vi "State_Waiting.vi"(8 "error in (no error)":T1, 9 "Parameter":variant, 10 "Command":string, 11 "Sim DiscreteIO in":class) -> (0 "error out":T1, 2 "Debug Message":string, 3 "Sim DiscreteIO out":class)   [LabVIEW 2021, in "Sim DiscreteIO.lvclass"]
uses:
  Sim DiscreteIO.lvclass
  C:/Program Files (x86)/National Instruments/LabVIEW 2021/user.lib/S2 Labs/Module Framework/Modules/Base/Module.lvclass
  Sim DiscreteIO.lvclass/Sim DiscreteIO.ctl
  <userlib>/S2 Labs/Module Framework/Modules/Base/Module.lvclass/Module.ctl
  <userlib>/S2 Labs/CVT Toolkit/CVT.lvclass/CVT.ctl
  c5649ace-d903-4788-aea9-226f7769309e.vi
  82162073-8ea0-43ea-a5e7-9bcd401e2448.vi
  Accessors/Write Initialized.vi
  Accessors/Read ch_labels.vi
  Accessors/Read occurrence.vi
  82162073-8ea0-43ea-a5e7-9bcd401e2448.vi/71b19a30-41bb-452f-8775-2cd3e07414b9.vi
  <userlib>/S2 Labs/Module Framework/Modules/Base/Read Module CVT.vi
  <userlib>/S2 Labs/CVT Toolkit/Variant Functions/Write Reserved Attributes.vi
  <userlib>/S2 Labs/CVT Toolkit/Read CVT DVR.vi
  <userlib>/S2 Labs/CVT Toolkit/Variant Functions/Write Alias Attribute.vi
  <userlib>/S2 Labs/CVT Toolkit/Variant Functions/Write Unit Attribute.vi
  <userlib>/S2 Labs/CVT Toolkit/Variant Functions/Write Type Attribute.vi
  <userlib>/S2 Labs/CVT Toolkit/Variant Functions/Write Parms Attribute.vi
  <vilib>/Utility/error.llb/Error Cluster From Error Code.vi
  <vilib>/rvi/errors/niLvFpgaAdjustHostInterfaceError.vi
  <userlib>/S2 Labs/Module Framework/Modules/Base/Trigger Logging Write.vi
  <vilib>/rvi/interface/nirviReadWriteControl/nirviReadWriteControl.xnode
  <userlib>/S2 Labs/CVT Toolkit/CVT.lvclass
  <userlib>/S2 Labs/Module Framework/Modules/Base/Module.lvclass
  NiFpgaLv.dll
  <vilib>/rvi/interface/Simulation/niFpgaSimulationCallBeginRW.vi
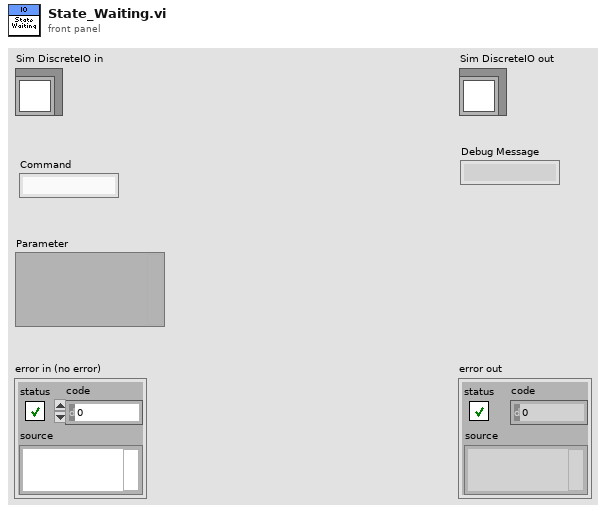
[diagram p1: front panel]
types:
  T1 = cluster{"source":string, "code":numeric, "status":boolean}
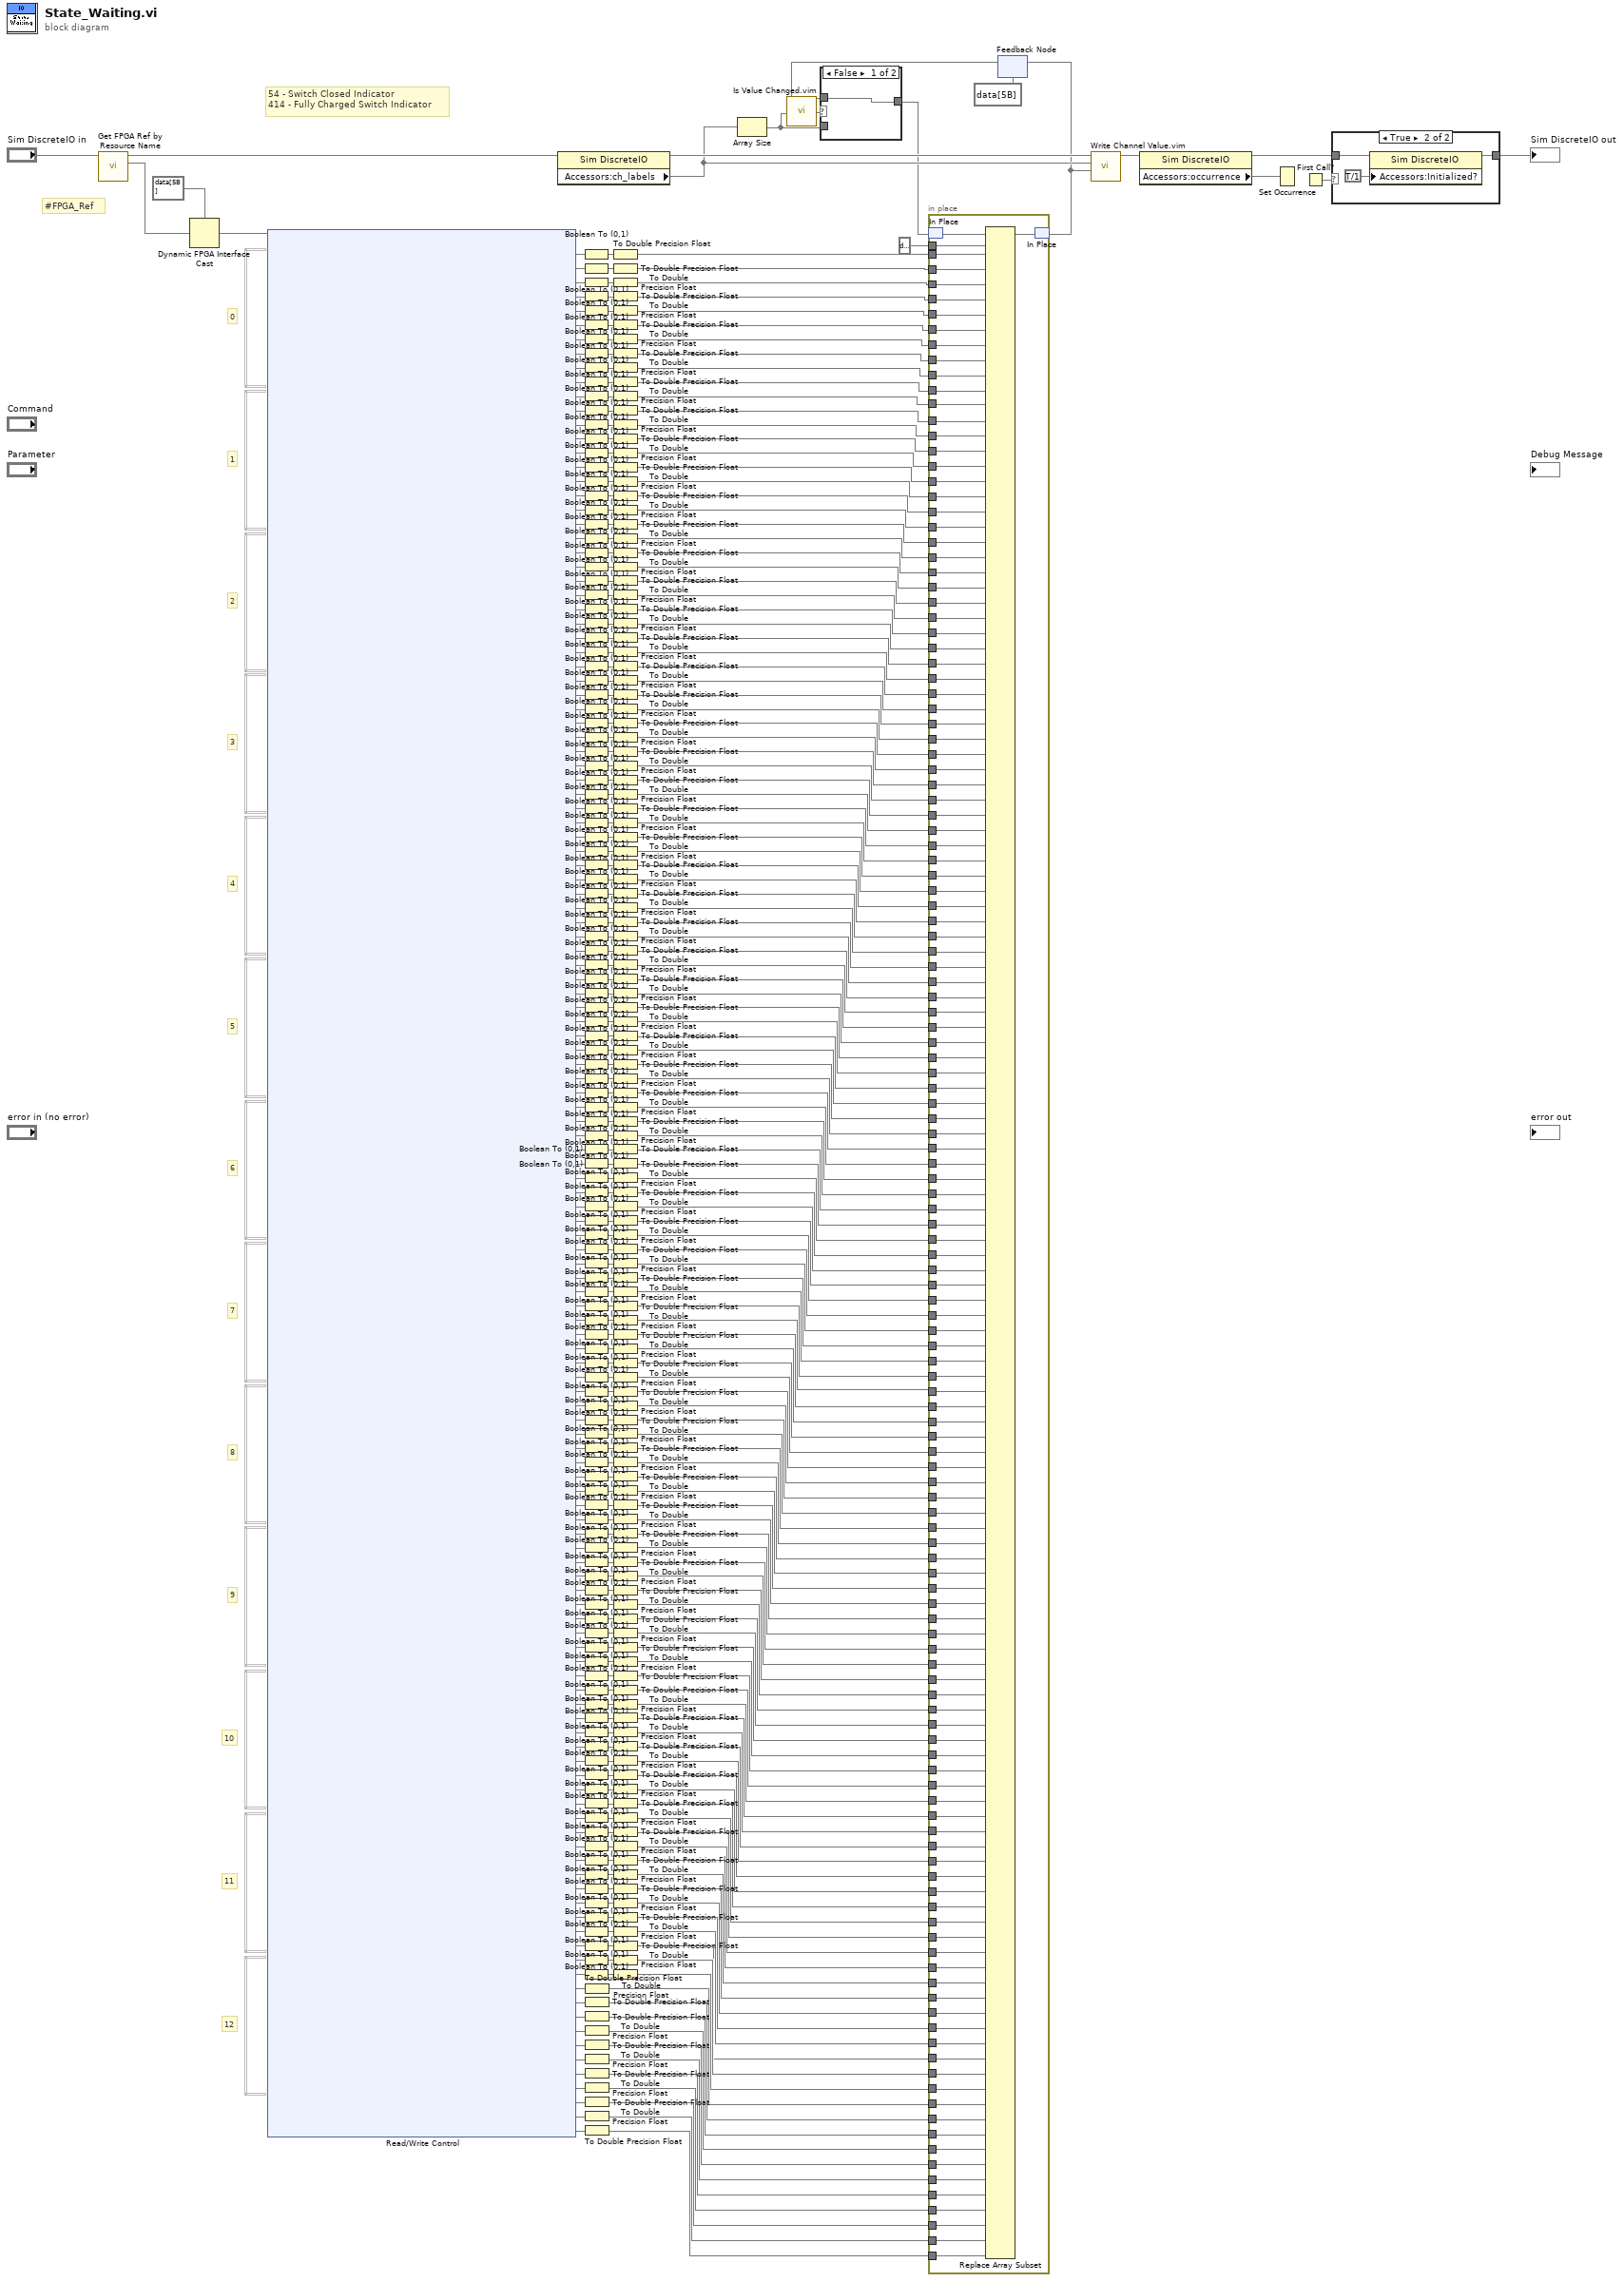
[diagram p0: block diagram]
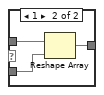
[diagram p2: hidden frame]
diagram:
  # "54 - Switch Closed Indicator\n414 - Fully Charged Switch Indicator"
  # "12"
  # "11"
  # "10"
  # "9"
  # "8"
  # "7"
  # "6"
  # "5"
  # "4"
  # "3"
  # "2"
  # "1"
  # "0"
  # "#FPGA_Ref"
  n1 = call <userlib>:"Get FPGA Ref by Resource Name.vi"(11:"Sim DiscreteIO in") -> (2:w405, 3:w12)  [unwired: 7 in, 2 out]
  n2 = Dynamic FPGA Interface Cast(Session In=data[5B] ("Type"), Type=w405) -> (Session Out=w17)
  n3 = xnode "Read/Write Control"(w17) -> (w20, w23, w26, w30, w35, w36, w37, w38, w44, w45, w57, w58, w59, w60, w61, w62, w63, w64, w65, w66, w86, w87, w88, w89, w90, w91, w92, w93, w94, w95, w115, w116, w117, w118, w119, w120, w121, w122, w123, w124, w148, w149, w150, w151, w152, w153, w154, w155, w156, w157, w178, w179, w180, w181, w182, w183, w184, w185, w186, w327, w328, w5, w4, w187, w208, w209, w210, w211, w212, w213, w214, w215, w216, w217, w238, w239, w240, w241, w242, w243, w244, w245, w246, w247, w267, w269, w270, w271, w272, w273, w274, w275, w276, w277, w296, w301, w302, w303, w330, w331, w304, w305, w333, w306, w307, w334, w345, w346, w351, w352, w357, w358, w364, w365, w366, w367, w379, w380, w381, w382, w383, w384, w312, w313, w314, w315, w316, w317, w318, w319, w320, w321, w322)  [unwired: 1 in, 2 out]
  n4 = property class="Sim DiscreteIO"(reference=w12) -> (reference out=w11, "Accessors:ch_labels"=w10)  [unwired: 1 in, 1 out]
  n5 = Boolean To (0,1)(Boolean=w20) -> (0, 1=w19)
  n6 = Boolean To (0,1)(Boolean=w23) -> (0, 1=w22)
  n7 = Boolean To (0,1)(Boolean=w26) -> (0, 1=w25)
  n8 = Boolean To (0,1)(Boolean=w30) -> (0, 1=w24)
  n9 = Boolean To (0,1)(Boolean=w35) -> (0, 1=w34)
  n10 = Boolean To (0,1)(Boolean=w36) -> (0, 1=w33)
  n11 = Boolean To (0,1)(Boolean=w37) -> (0, 1=w31)
  n12 = Boolean To (0,1)(Boolean=w38) -> (0, 1=w32)
  n13 = Boolean To (0,1)(Boolean=w44) -> (0, 1=w133)
  n14 = Boolean To (0,1)(Boolean=w45) -> (0, 1=w43)
  n15 = Boolean To (0,1)(Boolean=w57) -> (0, 1=w56)
  n16 = Boolean To (0,1)(Boolean=w58) -> (0, 1=w55)
  n17 = Boolean To (0,1)(Boolean=w59) -> (0, 1=w53)
  n18 = Boolean To (0,1)(Boolean=w60) -> (0, 1=w54)
  n19 = Boolean To (0,1)(Boolean=w61) -> (0, 1=w49)
  n20 = Boolean To (0,1)(Boolean=w62) -> (0, 1=w50)
  n21 = Boolean To (0,1)(Boolean=w63) -> (0, 1=w52)
  n22 = Boolean To (0,1)(Boolean=w64) -> (0, 1=w51)
  n23 = Boolean To (0,1)(Boolean=w65) -> (0, 1=w324)
  n24 = Boolean To (0,1)(Boolean=w66) -> (0, 1=w48)
  n25 = Boolean To (0,1)(Boolean=w86) -> (0, 1=w77)
  n26 = Boolean To (0,1)(Boolean=w87) -> (0, 1=w78)
  n27 = Boolean To (0,1)(Boolean=w88) -> (0, 1=w80)
  n28 = Boolean To (0,1)(Boolean=w89) -> (0, 1=w79)
  n29 = Boolean To (0,1)(Boolean=w90) -> (0, 1=w84)
  n30 = Boolean To (0,1)(Boolean=w91) -> (0, 1=w83)
  n31 = Boolean To (0,1)(Boolean=w92) -> (0, 1=w81)
  n32 = Boolean To (0,1)(Boolean=w93) -> (0, 1=w82)
  n33 = Boolean To (0,1)(Boolean=w94) -> (0, 1=w132)
  n34 = Boolean To (0,1)(Boolean=w95) -> (0, 1=w85)
  n35 = Boolean To (0,1)(Boolean=w115) -> (0, 1=w114)
  n36 = Boolean To (0,1)(Boolean=w116) -> (0, 1=w113)
  n37 = Boolean To (0,1)(Boolean=w117) -> (0, 1=w111)
  n38 = Boolean To (0,1)(Boolean=w118) -> (0, 1=w112)
  n39 = Boolean To (0,1)(Boolean=w119) -> (0, 1=w107)
  n40 = Boolean To (0,1)(Boolean=w120) -> (0, 1=w108)
  n41 = Boolean To (0,1)(Boolean=w121) -> (0, 1=w110)
  n42 = Boolean To (0,1)(Boolean=w122) -> (0, 1=w109)
  n43 = Boolean To (0,1)(Boolean=w123) -> (0, 1=w131)
  n44 = Boolean To (0,1)(Boolean=w124) -> (0, 1=w106)
  n45 = Boolean To (0,1)(Boolean=w148) -> (0, 1=w139)
  n46 = Boolean To (0,1)(Boolean=w149) -> (0, 1=w140)
  n47 = Boolean To (0,1)(Boolean=w150) -> (0, 1=w142)
  n48 = Boolean To (0,1)(Boolean=w151) -> (0, 1=w141)
  n49 = Boolean To (0,1)(Boolean=w152) -> (0, 1=w146)
  n50 = Boolean To (0,1)(Boolean=w153) -> (0, 1=w145)
  n51 = Boolean To (0,1)(Boolean=w154) -> (0, 1=w143)
  n52 = Boolean To (0,1)(Boolean=w155) -> (0, 1=w144)
  n53 = Boolean To (0,1)(Boolean=w156) -> (0, 1=w138)
  n54 = Boolean To (0,1)(Boolean=w157) -> (0, 1=w147)
  n55 = Boolean To (0,1)(Boolean=w178) -> (0, 1=w176)
  n56 = Boolean To (0,1)(Boolean=w179) -> (0, 1=w175)
  n57 = Boolean To (0,1)(Boolean=w180) -> (0, 1=w173)
  n58 = Boolean To (0,1)(Boolean=w181) -> (0, 1=w174)
  n59 = Boolean To (0,1)(Boolean=w182) -> (0, 1=w169)
  n60 = Boolean To (0,1)(Boolean=w183) -> (0, 1=w170)
  n61 = Boolean To (0,1)(Boolean=w184) -> (0, 1=w172)
  n62 = Boolean To (0,1)(Boolean=w185) -> (0, 1=w171)
  n63 = Boolean To (0,1)(Boolean=w186) -> (0, 1=w177)
  n64 = Boolean To (0,1)(Boolean=w327) -> (0, 1=w326)
  n65 = Boolean To (0,1)(Boolean=w328) -> (0, 1=w325)
  n66 = Boolean To (0,1)(Boolean=w5) -> (0, 1=w6)
  n67 = Boolean To (0,1)(Boolean=w4) -> (0, 1=w7)
  n68 = Boolean To (0,1)(Boolean=w187) -> (0, 1=w168)
  n69 = Boolean To (0,1)(Boolean=w208) -> (0, 1=w199)
  n70 = Boolean To (0,1)(Boolean=w209) -> (0, 1=w200)
  n71 = Boolean To (0,1)(Boolean=w210) -> (0, 1=w202)
  n72 = Boolean To (0,1)(Boolean=w211) -> (0, 1=w201)
  n73 = Boolean To (0,1)(Boolean=w212) -> (0, 1=w206)
  n74 = Boolean To (0,1)(Boolean=w213) -> (0, 1=w205)
  n75 = Boolean To (0,1)(Boolean=w214) -> (0, 1=w203)
  n76 = Boolean To (0,1)(Boolean=w215) -> (0, 1=w204)
  n77 = Boolean To (0,1)(Boolean=w216) -> (0, 1=w198)
  n78 = Boolean To (0,1)(Boolean=w217) -> (0, 1=w207)
  n79 = Boolean To (0,1)(Boolean=w238) -> (0, 1=w236)
  n80 = Boolean To (0,1)(Boolean=w239) -> (0, 1=w235)
  n81 = Boolean To (0,1)(Boolean=w240) -> (0, 1=w233)
  n82 = Boolean To (0,1)(Boolean=w241) -> (0, 1=w234)
  n83 = Boolean To (0,1)(Boolean=w242) -> (0, 1=w229)
  n84 = Boolean To (0,1)(Boolean=w243) -> (0, 1=w230)
  n85 = Boolean To (0,1)(Boolean=w244) -> (0, 1=w232)
  n86 = Boolean To (0,1)(Boolean=w245) -> (0, 1=w231)
  n87 = Boolean To (0,1)(Boolean=w246) -> (0, 1=w237)
  n88 = Boolean To (0,1)(Boolean=w247) -> (0, 1=w228)
  n89 = Boolean To (0,1)(Boolean=w267) -> (0, 1=w268)
  n90 = Boolean To (0,1)(Boolean=w269) -> (0, 1=w259)
  n91 = Boolean To (0,1)(Boolean=w270) -> (0, 1=w261)
  n92 = Boolean To (0,1)(Boolean=w271) -> (0, 1=w260)
  n93 = Boolean To (0,1)(Boolean=w272) -> (0, 1=w265)
  n94 = Boolean To (0,1)(Boolean=w273) -> (0, 1=w264)
  n95 = Boolean To (0,1)(Boolean=w274) -> (0, 1=w262)
  n96 = Boolean To (0,1)(Boolean=w275) -> (0, 1=w263)
  n97 = Boolean To (0,1)(Boolean=w276) -> (0, 1=w258)
  n98 = Boolean To (0,1)(Boolean=w277) -> (0, 1=w266)
  n99 = Boolean To (0,1)(Boolean=w296) -> (0, 1=w288)
  n100 = Boolean To (0,1)(Boolean=w301) -> (0, 1=w294)
  n101 = Boolean To (0,1)(Boolean=w302) -> (0, 1=w292)
  n102 = Boolean To (0,1)(Boolean=w303) -> (0, 1=w293)
  n103 = Boolean To (0,1)(Boolean=w330) -> (0, 1=w329)
  n104 = Boolean To (0,1)(Boolean=w331) -> (0, 1=w341)
  n105 = Boolean To (0,1)(Boolean=w304) -> (0, 1=w290)
  n106 = Boolean To (0,1)(Boolean=w305) -> (0, 1=w291)
  n107 = Boolean To (0,1)(Boolean=w333) -> (0, 1=w332)
  n108 = Boolean To (0,1)(Boolean=w306) -> (0, 1=w295)
  n109 = Boolean To (0,1)(Boolean=w307) -> (0, 1=w289)
  n110 = Boolean To (0,1)(Boolean=w334) -> (0, 1=w342)
  n111 = Boolean To (0,1)(Boolean=w345) -> (0, 1=w344)
  n112 = Boolean To (0,1)(Boolean=w346) -> (0, 1=w343)
  n113 = Boolean To (0,1)(Boolean=w351) -> (0, 1=w349)
  n114 = Boolean To (0,1)(Boolean=w352) -> (0, 1=w350)
  n115 = Boolean To (0,1)(Boolean=w357) -> (0, 1=w356)
  n116 = Boolean To (0,1)(Boolean=w358) -> (0, 1=w355)
  n117 = Boolean To (0,1)(Boolean=w364) -> (0, 1=w372)
  n118 = Boolean To (0,1)(Boolean=w365) -> (0, 1=w363)
  n119 = Boolean To (0,1)(Boolean=w366) -> (0, 1=w361)
  n120 = Boolean To (0,1)(Boolean=w367) -> (0, 1=w362)
  n121 = Boolean To (0,1)(Boolean=w379) -> (0, 1=w377)
  n122 = Boolean To (0,1)(Boolean=w380) -> (0, 1=w378)
  n123 = Boolean To (0,1)(Boolean=w381) -> (0, 1=w373)
  n124 = Boolean To (0,1)(Boolean=w382) -> (0, 1=w374)
  n125 = Boolean To (0,1)(Boolean=w383) -> (0, 1=w376)
  n126 = Boolean To (0,1)(Boolean=w384) -> (0, 1=w375)
  n127 = To Double Precision Float(number=w312) -> (double precision float=w391)
  n128 = To Double Precision Float(number=w313) -> (double precision float=w392)
  n129 = To Double Precision Float(number=w314) -> (double precision float=w393)
  n130 = To Double Precision Float(number=w315) -> (double precision float=w394)
  n131 = To Double Precision Float(number=w316) -> (double precision float=w395)
  n132 = To Double Precision Float(number=w317) -> (double precision float=w396)
  n133 = To Double Precision Float(number=w318) -> (double precision float=w397)
  n134 = To Double Precision Float(number=w319) -> (double precision float=w398)
  n135 = To Double Precision Float(number=w320) -> (double precision float=w399)
  n136 = To Double Precision Float(number=w321) -> (double precision float=w1)
  n137 = To Double Precision Float(number=w322) -> (double precision float=w323)
  n138 = To Double Precision Float(number=w19) -> (double precision float=w21)
  n139 = To Double Precision Float(number=w22) -> (double precision float=w27)
  n140 = To Double Precision Float(number=w25) -> (double precision float=w28)
  n141 = To Double Precision Float(number=w24) -> (double precision float=w29)
  n142 = To Double Precision Float(number=w34) -> (double precision float=w39)
  n143 = To Double Precision Float(number=w33) -> (double precision float=w40)
  n144 = To Double Precision Float(number=w31) -> (double precision float=w41)
  n145 = To Double Precision Float(number=w32) -> (double precision float=w42)
  n146 = To Double Precision Float(number=w133) -> (double precision float=w46)
  n147 = To Double Precision Float(number=w43) -> (double precision float=w47)
  n148 = To Double Precision Float(number=w56) -> (double precision float=w67)
  n149 = To Double Precision Float(number=w55) -> (double precision float=w68)
  n150 = To Double Precision Float(number=w53) -> (double precision float=w69)
  n151 = To Double Precision Float(number=w54) -> (double precision float=w70)
  n152 = To Double Precision Float(number=w49) -> (double precision float=w71)
  n153 = To Double Precision Float(number=w50) -> (double precision float=w72)
  n154 = To Double Precision Float(number=w52) -> (double precision float=w73)
  n155 = To Double Precision Float(number=w51) -> (double precision float=w74)
  n156 = To Double Precision Float(number=w324) -> (double precision float=w75)
  n157 = To Double Precision Float(number=w48) -> (double precision float=w76)
  n158 = To Double Precision Float(number=w77) -> (double precision float=w96)
  n159 = To Double Precision Float(number=w78) -> (double precision float=w97)
  n160 = To Double Precision Float(number=w80) -> (double precision float=w98)
  n161 = To Double Precision Float(number=w79) -> (double precision float=w99)
  n162 = To Double Precision Float(number=w84) -> (double precision float=w100)
  n163 = To Double Precision Float(number=w83) -> (double precision float=w101)
  n164 = To Double Precision Float(number=w81) -> (double precision float=w102)
  n165 = To Double Precision Float(number=w82) -> (double precision float=w103)
  n166 = To Double Precision Float(number=w132) -> (double precision float=w104)
  n167 = To Double Precision Float(number=w85) -> (double precision float=w105)
  n168 = To Double Precision Float(number=w114) -> (double precision float=w125)
  n169 = To Double Precision Float(number=w113) -> (double precision float=w126)
  n170 = To Double Precision Float(number=w111) -> (double precision float=w127)
  n171 = To Double Precision Float(number=w112) -> (double precision float=w128)
  n172 = To Double Precision Float(number=w107) -> (double precision float=w129)
  n173 = To Double Precision Float(number=w108) -> (double precision float=w130)
  n174 = To Double Precision Float(number=w110) -> (double precision float=w134)
  n175 = To Double Precision Float(number=w109) -> (double precision float=w135)
  n176 = To Double Precision Float(number=w131) -> (double precision float=w136)
  n177 = To Double Precision Float(number=w106) -> (double precision float=w137)
  n178 = To Double Precision Float(number=w139) -> (double precision float=w158)
  n179 = To Double Precision Float(number=w140) -> (double precision float=w159)
  n180 = To Double Precision Float(number=w142) -> (double precision float=w160)
  n181 = To Double Precision Float(number=w141) -> (double precision float=w161)
  n182 = To Double Precision Float(number=w146) -> (double precision float=w162)
  n183 = To Double Precision Float(number=w145) -> (double precision float=w163)
  n184 = To Double Precision Float(number=w143) -> (double precision float=w164)
  n185 = To Double Precision Float(number=w144) -> (double precision float=w165)
  n186 = To Double Precision Float(number=w138) -> (double precision float=w166)
  n187 = To Double Precision Float(number=w147) -> (double precision float=w167)
  n188 = To Double Precision Float(number=w176) -> (double precision float=w188)
  n189 = To Double Precision Float(number=w175) -> (double precision float=w189)
  n190 = To Double Precision Float(number=w173) -> (double precision float=w190)
  n191 = To Double Precision Float(number=w174) -> (double precision float=w191)
  n192 = To Double Precision Float(number=w169) -> (double precision float=w192)
  n193 = To Double Precision Float(number=w170) -> (double precision float=w193)
  n194 = To Double Precision Float(number=w172) -> (double precision float=w194)
  n195 = To Double Precision Float(number=w171) -> (double precision float=w195)
  n196 = To Double Precision Float(number=w177) -> (double precision float=w196)
  n197 = To Double Precision Float(number=w326) -> (double precision float=w339)
  n198 = To Double Precision Float(number=w325) -> (double precision float=w340)
  n199 = To Double Precision Float(number=w6) -> (double precision float=w3)
  n200 = To Double Precision Float(number=w7) -> (double precision float=w2)
  n201 = To Double Precision Float(number=w168) -> (double precision float=w197)
  n202 = To Double Precision Float(number=w199) -> (double precision float=w218)
  n203 = To Double Precision Float(number=w200) -> (double precision float=w219)
  n204 = To Double Precision Float(number=w202) -> (double precision float=w220)
  n205 = To Double Precision Float(number=w201) -> (double precision float=w221)
  n206 = To Double Precision Float(number=w206) -> (double precision float=w222)
  n207 = To Double Precision Float(number=w205) -> (double precision float=w223)
  n208 = To Double Precision Float(number=w203) -> (double precision float=w224)
  n209 = To Double Precision Float(number=w204) -> (double precision float=w225)
  n210 = To Double Precision Float(number=w198) -> (double precision float=w226)
  n211 = To Double Precision Float(number=w207) -> (double precision float=w227)
  n212 = To Double Precision Float(number=w236) -> (double precision float=w248)
  n213 = To Double Precision Float(number=w235) -> (double precision float=w249)
  n214 = To Double Precision Float(number=w233) -> (double precision float=w250)
  n215 = To Double Precision Float(number=w234) -> (double precision float=w251)
  n216 = To Double Precision Float(number=w229) -> (double precision float=w252)
  n217 = To Double Precision Float(number=w230) -> (double precision float=w253)
  n218 = To Double Precision Float(number=w232) -> (double precision float=w254)
  n219 = To Double Precision Float(number=w231) -> (double precision float=w255)
  n220 = To Double Precision Float(number=w237) -> (double precision float=w256)
  n221 = To Double Precision Float(number=w228) -> (double precision float=w257)
  n222 = To Double Precision Float(number=w268) -> (double precision float=w278)
  n223 = To Double Precision Float(number=w259) -> (double precision float=w279)
  n224 = To Double Precision Float(number=w261) -> (double precision float=w280)
  n225 = To Double Precision Float(number=w260) -> (double precision float=w281)
  n226 = To Double Precision Float(number=w265) -> (double precision float=w282)
  n227 = To Double Precision Float(number=w264) -> (double precision float=w283)
  n228 = To Double Precision Float(number=w262) -> (double precision float=w284)
  n229 = To Double Precision Float(number=w263) -> (double precision float=w285)
  n230 = To Double Precision Float(number=w258) -> (double precision float=w286)
  n231 = To Double Precision Float(number=w266) -> (double precision float=w287)
  n232 = To Double Precision Float(number=w288) -> (double precision float=w297)
  n233 = To Double Precision Float(number=w294) -> (double precision float=w298)
  n234 = To Double Precision Float(number=w292) -> (double precision float=w299)
  n235 = To Double Precision Float(number=w293) -> (double precision float=w300)
  n236 = To Double Precision Float(number=w329) -> (double precision float=w337)
  n237 = To Double Precision Float(number=w341) -> (double precision float=w338)
  n238 = To Double Precision Float(number=w290) -> (double precision float=w308)
  n239 = To Double Precision Float(number=w291) -> (double precision float=w309)
  n240 = To Double Precision Float(number=w332) -> (double precision float=w336)
  n241 = To Double Precision Float(number=w295) -> (double precision float=w310)
  n242 = To Double Precision Float(number=w289) -> (double precision float=w311)
  n243 = To Double Precision Float(number=w342) -> (double precision float=w335)
  n244 = To Double Precision Float(number=w344) -> (double precision float=w347)
  n245 = To Double Precision Float(number=w343) -> (double precision float=w348)
  n246 = To Double Precision Float(number=w349) -> (double precision float=w353)
  n247 = To Double Precision Float(number=w350) -> (double precision float=w354)
  n248 = To Double Precision Float(number=w356) -> (double precision float=w359)
  n249 = To Double Precision Float(number=w355) -> (double precision float=w360)
  n250 = To Double Precision Float(number=w372) -> (double precision float=w368)
  n251 = To Double Precision Float(number=w363) -> (double precision float=w369)
  n252 = To Double Precision Float(number=w361) -> (double precision float=w370)
  n253 = To Double Precision Float(number=w362) -> (double precision float=w371)
  n254 = To Double Precision Float(number=w377) -> (double precision float=w385)
  n255 = To Double Precision Float(number=w378) -> (double precision float=w386)
  n256 = To Double Precision Float(number=w373) -> (double precision float=w387)
  n257 = To Double Precision Float(number=w374) -> (double precision float=w388)
  n258 = To Double Precision Float(number=w376) -> (double precision float=w389)
  n259 = To Double Precision Float(number=w375) -> (double precision float=w390)
  n260 = Array Size(array=w10) -> (size(s)=w14)
  n261 = call "Is Value Changed.vim"(1:w14) -> (0:w16)
  n262 = feedback #1(data[5B]) -> (w15)
  n263 = case shown="False" w16 {
    tunnel: w14 -> [_ w409]
    tunnel: [w408 w410] -> w9
    tunnel: w15 -> [w408 w411]
    frame 0 {
    }
    frame 1 {
      n264 = Reshape Array(w411, w409) -> (w410)
    }
  }
  n265 = in-place {
    in-place-border: data[5B] ("index") -> [w547]
    in-place-border: w21 -> [w546]
    in-place-border: w27 -> [w545]
    in-place-border: w28 -> [w544]
    in-place-border: w29 -> [w543]
    in-place-border: w39 -> [w542]
    in-place-border: w40 -> [w541]
    in-place-border: w41 -> [w540]
    in-place-border: w42 -> [w539]
    in-place-border: w46 -> [w532]
    in-place-border: w47 -> [w531]
    in-place-border: w68 -> [w538]
    in-place-border: w69 -> [w537]
    in-place-border: w70 -> [w536]
    in-place-border: w71 -> [w535]
    in-place-border: w67 -> [w530]
    in-place-border: w72 -> [w529]
    in-place-border: w73 -> [w528]
    in-place-border: w74 -> [w527]
    in-place-border: w75 -> [w526]
    in-place-border: w76 -> [w525]
    in-place-border: w96 -> [w524]
    in-place-border: w97 -> [w523]
    in-place-border: w98 -> [w522]
    in-place-border: w99 -> [w521]
    in-place-border: w100 -> [w520]
    in-place-border: w101 -> [w519]
    in-place-border: w102 -> [w518]
    in-place-border: w103 -> [w517]
    in-place-border: w104 -> [w516]
    in-place-border: w105 -> [w515]
    in-place-border: w125 -> [w514]
    in-place-border: w126 -> [w513]
    in-place-border: w127 -> [w512]
    in-place-border: w128 -> [w511]
    in-place-border: w129 -> [w510]
    in-place-border: w130 -> [w509]
    in-place-border: w134 -> [w508]
    in-place-border: w135 -> [w507]
    in-place-border: w136 -> [w506]
    in-place-border: w137 -> [w505]
    in-place-border: w158 -> [w504]
    in-place-border: w159 -> [w503]
    in-place-border: w160 -> [w502]
    in-place-border: w161 -> [w501]
    in-place-border: w162 -> [w500]
    in-place-border: w163 -> [w499]
    in-place-border: w164 -> [w498]
    in-place-border: w165 -> [w497]
    in-place-border: w166 -> [w496]
    in-place-border: w167 -> [w495]
    in-place-border: w188 -> [w494]
    in-place-border: w189 -> [w493]
    in-place-border: w190 -> [w492]
    in-place-border: w191 -> [w491]
    in-place-border: w192 -> [w490]
    in-place-border: w193 -> [w489]
    in-place-border: w194 -> [w488]
    in-place-border: w195 -> [w487]
    in-place-border: w196 -> [w486]
    in-place-border: w197 -> [w439]
    in-place-border: w219 -> [w441]
    in-place-border: w220 -> [w442]
    in-place-border: w221 -> [w443]
    in-place-border: w222 -> [w444]
    in-place-border: w223 -> [w445]
    in-place-border: w224 -> [w446]
    in-place-border: w225 -> [w447]
    in-place-border: w226 -> [w448]
    in-place-border: w227 -> [w449]
    in-place-border: w248 -> [w450]
    in-place-border: w249 -> [w451]
    in-place-border: w250 -> [w452]
    in-place-border: w251 -> [w453]
    in-place-border: w252 -> [w454]
    in-place-border: w253 -> [w455]
    in-place-border: w254 -> [w456]
    in-place-border: w255 -> [w457]
    in-place-border: w256 -> [w458]
    in-place-border: w300 -> [w473]
    in-place-border: w218 -> [w440]
    in-place-border: w257 -> [w459]
    in-place-border: w278 -> [w460]
    in-place-border: w281 -> [w463]
    in-place-border: w282 -> [w464]
    in-place-border: w279 -> [w461]
    in-place-border: w280 -> [w462]
    in-place-border: w287 -> [w469]
    in-place-border: w297 -> [w470]
    in-place-border: w298 -> [w471]
    in-place-border: w299 -> [w472]
    in-place-border: w283 -> [w465]
    in-place-border: w284 -> [w466]
    in-place-border: w285 -> [w467]
    in-place-border: w286 -> [w468]
    in-place-border: w308 -> [w476]
    in-place-border: w309 -> [w477]
    in-place-border: w310 -> [w479]
    in-place-border: w311 -> [w480]
    in-place-border: w391 -> [w418]
    in-place-border: w392 -> [w419]
    in-place-border: w393 -> [w420]
    in-place-border: w394 -> [w421]
    in-place-border: w395 -> [w422]
    in-place-border: w396 -> [w423]
    in-place-border: w397 -> [w424]
    in-place-border: w398 -> [w425]
    in-place-border: w399 -> [w426]
    in-place-border: w1 -> [w427]
    in-place-border: w323 -> [w428]
    in-place-border: w335 -> [w481]
    in-place-border: w336 -> [w478]
    in-place-border: w337 -> [w474]
    in-place-border: w338 -> [w475]
    in-place-border: w339 -> [w485]
    in-place-border: w340 -> [w484]
    in-place-border: w347 -> [w483]
    in-place-border: w348 -> [w482]
    in-place-border: w3 -> [w438]
    in-place-border: w2 -> [w437]
    in-place-border: w353 -> [w436]
    in-place-border: w354 -> [w435]
    in-place-border: w359 -> [w434]
    in-place-border: w360 -> [w433]
    in-place-border: w368 -> [w432]
    in-place-border: w369 -> [w431]
    in-place-border: w370 -> [w430]
    in-place-border: w371 -> [w429]
    in-place-border: w385 -> [w417]
    in-place-border: w386 -> [w416]
    in-place-border: w387 -> [w415]
    in-place-border: w388 -> [w414]
    in-place-border: w389 -> [w413]
    in-place-border: w390 -> [w412]
    n266 = in-place-match #2(w9) -> (w534)
    n267 = Replace Array Subset(array=w534, new element #1=w546, index #1=w547, new element #2=w545, new element #3=w544, new element #4=w543, new element #5=w542, new element #6=w541, new element #7=w540, new element #8=w539, new element #9=w532, new element #10=w531, new element #11=w530, new element #12=w538, new element #13=w537, new element #14=w536, new element #15=w535, new element #16=w529, new element #17=w528, new element #18=w527, new element #19=w526, new element #20=w525, new element #21=w524, new element #22=w523, new element #23=w522, new element #24=w521, new element #25=w520, new element #26=w519, new element #27=w518, new element #28=w517, new element #29=w516, new element #30=w515, new element #31=w514, new element #32=w513, new element #33=w512, new element #34=w511, new element #35=w510, new element #36=w509, new element #37=w508, new element #38=w507, new element #39=w506, new element #40=w505, new element #41=w504, new element #42=w503, new element #43=w502, new element #44=w501, new element #45=w500, new element #46=w499, new element #47=w498, new element #48=w497, new element #49=w496, new element #50=w495, new element #51=w494, new element #52=w493, new element #53=w492, new element #54=w491, new element #55=w490, new element #56=w489, new element #57=w488, new element #58=w487, new element #59=w486, new element #60=w485, new element #61=w484, new element #62=w438, new element #63=w437, new element #64=w439, new element #65=w440, new element #66=w441, new element #67=w442, new element #68=w443, new element #69=w444, new element #70=w445, new element #71=w446, new element #72=w447, new element #73=w448, new element #74=w449, new element #75=w450, new element #76=w451, new element #77=w452, new element #78=w453, new element #79=w454, new element #80=w455, new element #81=w456, new element #82=w457, new element #83=w458, new element #84=w459, new element #85=w460, new element #86=w461, new element #87=w462, new element #88=w463, new element #89=w464, new element #90=w465, new element #91=w466, new element #92=w467, new element #93=w468, new element #94=w469, new element #95=w470, new element #96=w471, new element #97=w472, new element #98=w473, new element #99=w474, new element #100=w475, new element #101=w476, new element #102=w477, new element #103=w478, new element #104=w479, new element #105=w480, new element #106=w481, new element #107=w483, new element #108=w482, new element #109=w436, new element #110=w435, new element #111=w434, new element #112=w433, new element #113=w432, new element #114=w431, new element #115=w430, new element #116=w429, new element #117=w417, new element #118=w416, new element #119=w415, new element #120=w414, new element #121=w413, new element #122=w412, new element #123=w418, new element #124=w419, new element #125=w420, new element #126=w421, new element #127=w422, new element #128=w423, new element #129=w424, new element #130=w425, new element #131=w426, new element #132=w427, new element #133=w428) -> (w533)  [unwired: 132 in]
    n268 = in-place-match #2(w533) -> (w8)
  }
  n269 = feedback-in #1(w8) -> ()
  n270 = call "Write Channel Value.vim"(9:w8, 10:w10, 11:w11) -> (3:w401)  [unwired: 6 in, 2 out]
  n271 = property class="Sim DiscreteIO"(reference=w401) -> (reference out=w400, "Accessors:occurrence"=w402)  [unwired: 1 in, 1 out]
  n272 = Set Occurrence(w402) -> ()
  n273 = First Call?() -> (First Call?: T/F=w403)
  n274 = case shown="True" w403 {
    tunnel: w400 -> [w548 w551]
    tunnel: [w548 w550] -> w404
    frame 0 {
    }
    frame 1 {
      n275 = property class="Sim DiscreteIO"(reference=w551, "Accessors:Initialized?"=T/1 ("Initialized?")) -> (reference out=w550)  [unwired: 1 in, 1 out]
    }
  }
  "Sim DiscreteIO out" <- w404
